vi "close.vi"(8 "error in (no error)":errorcluster, 11 "NI-9237 in":refnum<class "NI-9237.lvclass">) -> (0 "error out":errorcluster, 3 "NI-9237 out":refnum<class "NI-9237.lvclass">)   [LabVIEW 2025, in "Wheatstone Bridge.lvlib" / "NI-9237.lvclass"]
uses:
  NI-9237.lvclass
  NI-9237.lvclass/NI-9237.ctl
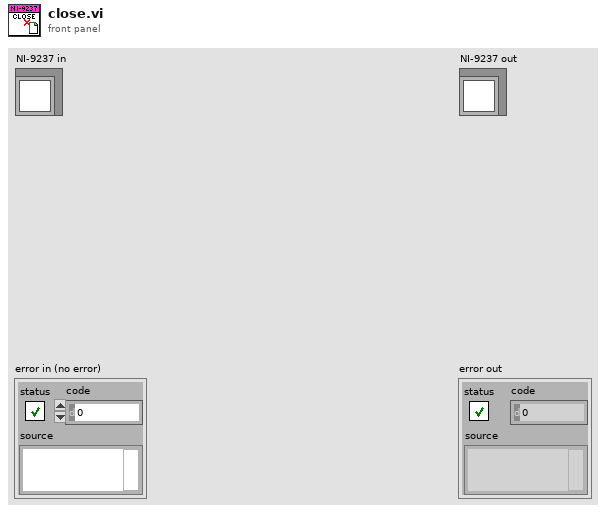
[diagram p1: front panel]
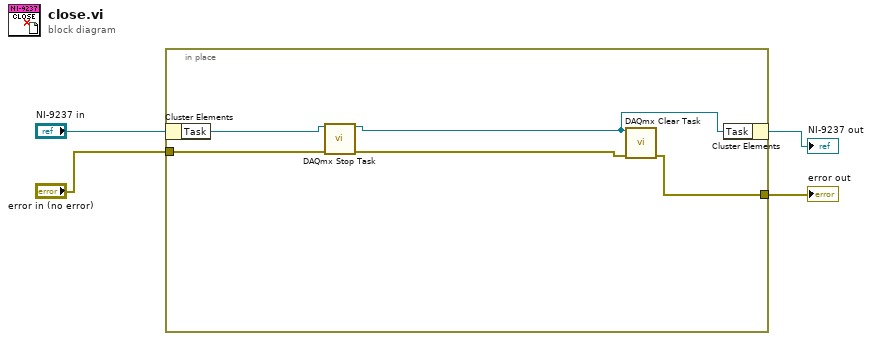
[diagram p0: block diagram]
diagram:
  n1 = in-place {
    in-place-border: [w9] -> w3
    in-place-border: "error in (no error)" -> [w5]
    n2 = in-place-cluster #1("NI-9237 in") -> ("Task"=w6:refnum<k21>)
    n3 = call <vilib>:"DAQmx Stop Task.vi"("task/channels in"=w6, "error in"=w5) -> ("task out"=w8:refnum<k21>, "error out"=w7:errorcluster)  [unwired: 12 in]
    n4 = call <vilib>:"DAQmx Clear Task.vi"("task in"=w8, "error in"=w7) -> ("error out"=w9:errorcluster)  [unwired: 13 in]
    n5 = in-place-cluster #1("Task"=w8) -> (→"NI-9237 out":refnum<class "NI-9237.lvclass">)
  }
  "error out" <- w3
